vi "TimerFGV.vi"(8 "error in (no error)":errorcluster, 10 "Target (s)":i32, 11 "Action":T1) -> (0 "error out":errorcluster, 2 "Elapsed":bool, 3 "Time":i32)   [LabVIEW 2017]
uses:
  TimerActionEnumControlFGV.ctl
  TimerInfoCluster.ctl
  TimerStateFGV.ctl
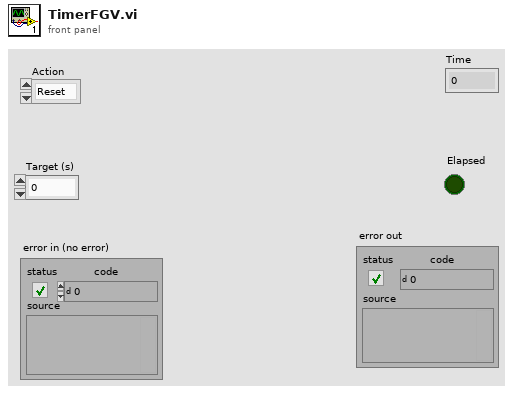
[diagram p1: front panel]
types:
  T1 = typedef "TimerActionEnumControlFGV.ctl" = enum16{"Reset", "TimeQuery", "Pause", "Unpause"}
  T2 = typedef "TimerInfoCluster.ctl" = cluster{"State":T3, "Elapsed":bool, "Target":u32, "Action":T1, "Last Time":timestamp, "Time":i32}
  T3 = typedef "TimerStateFGV.ctl" = enum16{"Reset", "Timing", "Paused", "Unpause"}
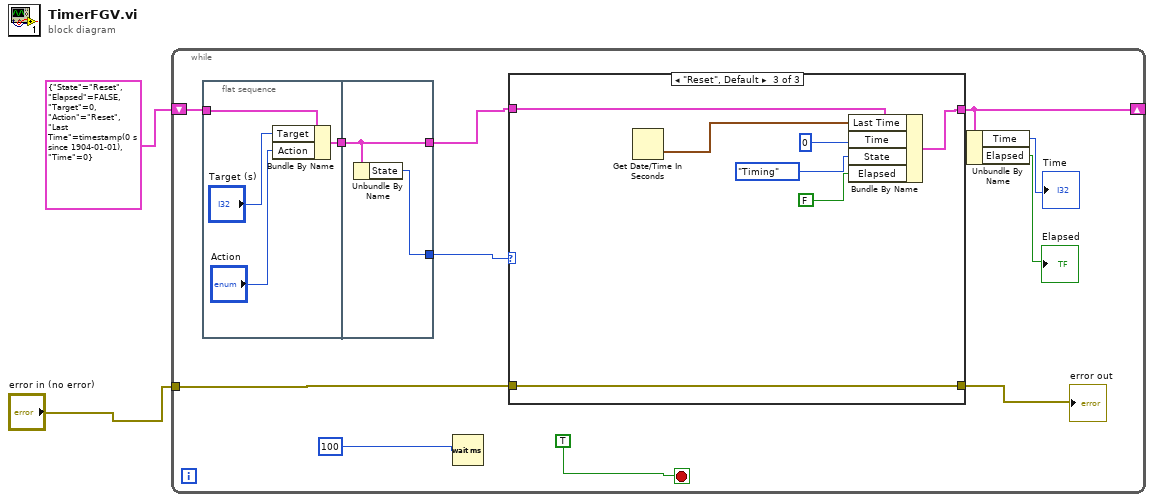
[diagram p0: block diagram]
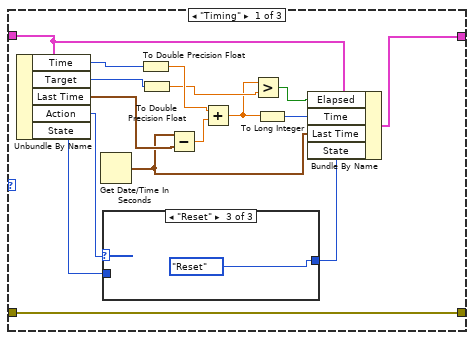
[diagram p2: hidden frame]
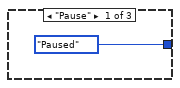
[diagram p3: hidden frame]
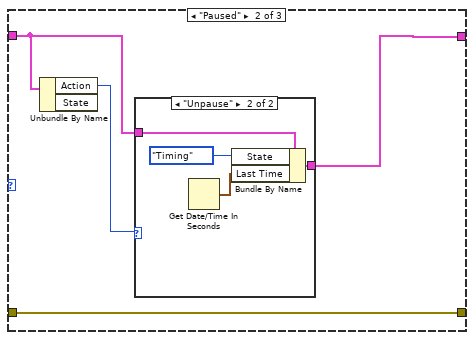
[diagram p5: hidden frame]
diagram:
  n1 = while {
    tunnel: "error in (no error)" -> [w11]
    shift-right: [w5] -> _
    shift-left: T2 {"State"=enum."Reset", "Elapsed"=FALSE, "Target"=0, "Action"=enum."Reset", "Last Time"=timestamp(0 s since 1904-01-01), "Time"=0} -> [w4]
    stop <- TRUE stop-if-true
    n2 = flat-sequence {
      tunnel: w4 -> [w17]
      tunnel: [w14] -> w7
      tunnel: [w19] -> w3
      tunnel: w7 -> [w19]
      tunnel: [w18] -> w6
      frame #0 {
        n3 = Bundle By Name(cluster=w17, "Target"="Target (s)", "Action"="Action") -> (w14:T2)
      }
      frame #1 {
        n4 = Unbundle By Name(w19) -> ("State"=w18:T3)
      }
    }
    n5 = Wait (ms)(milliseconds to wait=u32 100) -> ()  [unwired: 1 out]
    n6 = case shown="\"Reset\", Default" w6 {
      tunnel: w3 -> [w34 w41 w54]
      tunnel: w11 -> [w26 w39 w48]
      tunnel: [w32 w40 w49] -> w5
      tunnel: [w26 w39 w48] -> w8
      frame "Timing" {
        n7 = Unbundle By Name(w34) -> ("Time"=w25:i32, "Target"=w23:u32, "Last Time"=w35:timestamp, "Action"=w31:T1, "State"=w29:T3)
        n8 = Get Date/Time In Seconds() -> (seconds since 1Jan1904=w33:timestamp)
        n9 = case shown="\"Reset\"" w31 {
          tunnel: [TimerStateFGV."Paused" ("State") w37 TimerStateFGV."Reset" ("State")] -> w30
          tunnel: w29 -> [_ w37 _]
          frame "Pause" {
          }
          frame "TimeQuery", Default {
          }
          frame "Reset" {
          }
        }
        n10 = To Double Precision Float(number=w25) -> (double precision float=w24:dbl)
        n11 = To Double Precision Float(number=w23) -> (double precision float=w22:dbl)
        n12 = Subtract(x=w33, y=w35) -> (x-y=w27:dbl)
        n13 = Add(x=w24, y=w27) -> (x+y=w20:dbl)
        n14 = Greater?(x=w20, y=w22) -> (0:w28:bool)
        n15 = To Long Integer(number=w20) -> (32bit integer=w21:i32)
        n16 = Bundle By Name(cluster=w34, "Elapsed"=w28, "Time"=w21, "Last Time"=w33, "State"=w30) -> (w32:T2)
      }
      frame "Paused" {
        n17 = Unbundle By Name(w41) -> ("Action"=w42:T1)  [unwired: 1 out]
        n18 = case shown="\"Unpause\"" w42 {
          tunnel: w41 -> [w43 w47]
          tunnel: [w43 w44] -> w40
          frame "Pause", Default {
          }
          frame "Unpause" {
            n19 = Get Date/Time In Seconds() -> (seconds since 1Jan1904=w46:timestamp)
            n20 = Bundle By Name(cluster=w47, "State"=TimerStateFGV."Timing", "Last Time"=w46) -> (w44:T2)
          }
        }
      }
      frame "Reset", Default {
        n21 = Get Date/Time In Seconds() -> (seconds since 1Jan1904=w53:timestamp)
        n22 = Bundle By Name(cluster=w54, "Last Time"=w53, "Time"=0, "State"=TimerStateFGV."Timing", "Elapsed"=FALSE) -> (w49:T2)
      }
    }
    "error out" <- w8
    n23 = Unbundle By Name(w5) -> ("Time"=→"Time":i32, "Elapsed"=→"Elapsed":bool)
  }
